vi "Auto Set Arm Ramp.vi"(9 "Time (ms)":dbl, 10 "Arm Position":dbl, 11 "Run?":bool) -> (3 "Done":bool)   [LabVIEW 2013]
uses:
  Globals/Auto.vi
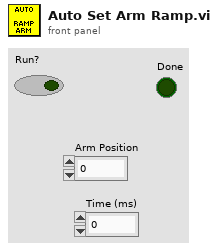
[diagram p1: front panel]
types:
  T1 = typedef "WPI_AnalogChannelDevRef.ctl" = cluster{"DevStatus":errorcluster, "Analog Module":T2, "Analog Channel":T3}
  T2 = typedef "FPGA_TypedefAnalogModule.ctl" = enum16{"Analog Module 1", "Analog Module 2"}
  T3 = typedef "FPGA_AIChannel.ctl" = enum8{"AI 1", "AI 2", "AI 3", "AI 4", "AI 5", "AI 6", "AI 7", "AI 8", "Invalid"}
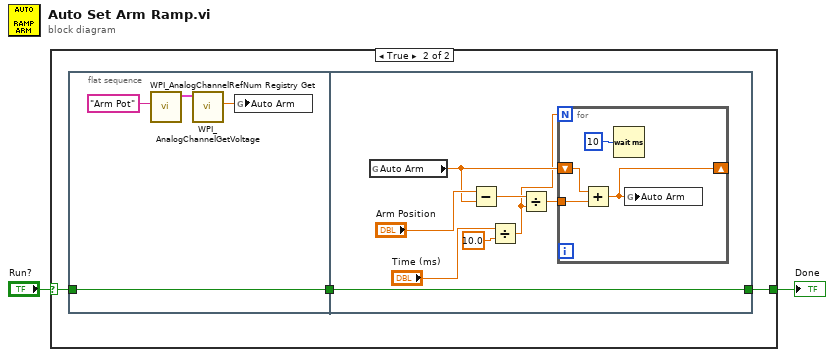
[diagram p0: block diagram]
diagram:
  n1 = case shown="True" "Run?" {
    selector: "Run?" -> [w3 w4]
    tunnel: [w3 w6] -> w1
    frame False {
    }
    frame True {
      n2 = flat-sequence {
        tunnel: [w10] -> w5
        tunnel: w4 -> [w10]
        tunnel: [w11] -> w6
        tunnel: w5 -> [w11]
        frame #0 {
          n3 = call <vilib>:"WPI_AnalogChannelRefNum Registry Get.vi"("refnum name"="Arm Pot") -> ("AIDeviceRef"=w9:T1)  [unwired: 9 in, 1 out]
          n4 = call <vilib>:"WPI_AnalogChannelGetVoltage.vi"("AIDeviceRef"=w9) -> ("Voltage"=w7:dbl)  [unwired: 8 in, 2 out]
          n5 = global write "Auto.vi" "Auto Arm"(w7) -> ()
        }
        frame #1 {
          n6 = global read "Auto.vi" "Auto Arm"() -> (w14:dbl)
          n7 = Subtract(x="Arm Position", y=w14) -> (x-y=w16:dbl)
          n8 = Divide(x="Time (ms)", y=10.0) -> (x/y=w12:dbl)
          n9 = Divide(x=w16, y=w12) -> (x/y=w13:dbl)
          n10 = for {
            N: w12 -> [_]
            shift-right: [w20] -> _
            shift-left: w14 -> [w21]
            tunnel: w13 -> [w19]
            n11 = Add(x=w21, y=w19) -> (x+y=w20:dbl)
            n12 = Wait (ms)(milliseconds to wait=u32 10) -> ()  [unwired: 1 out]
            n13 = global write "Auto.vi" "Auto Arm"(w20) -> ()
          }
        }
      }
    }
  }
  "Done" <- w1
